vi "读取dev setup.vi"() -> (3 "输出簇":T1)   [LabVIEW 2011]
uses:
  <vilib>/Utility/config.llb/Read Key (Double).vi
  <vilib>/Utility/config.llb/Read Key (String).vi
  <vilib>/Utility/config.llb/Write Key (Double).vi
  <vilib>/Utility/config.llb/Write Key (String).vi
  <vilib>/Utility/config.llb/NI_LVConfig.lvlib
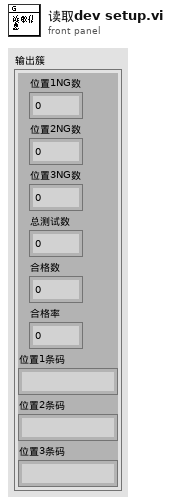
[diagram p1: front panel]
types:
  T1 = cluster{"位置1NG数 ":dbl, "位置2NG数 ":dbl, "位置3NG数 ":dbl, "总测试数":dbl, "合格数":dbl, "合格率":dbl, "位置1条码":string, "位置2条码":string, "位置3条码":string}
  T2 = typedef "NI_LVConfig.lvlib/Config Data RefNum.ctl" = refnum<k1>
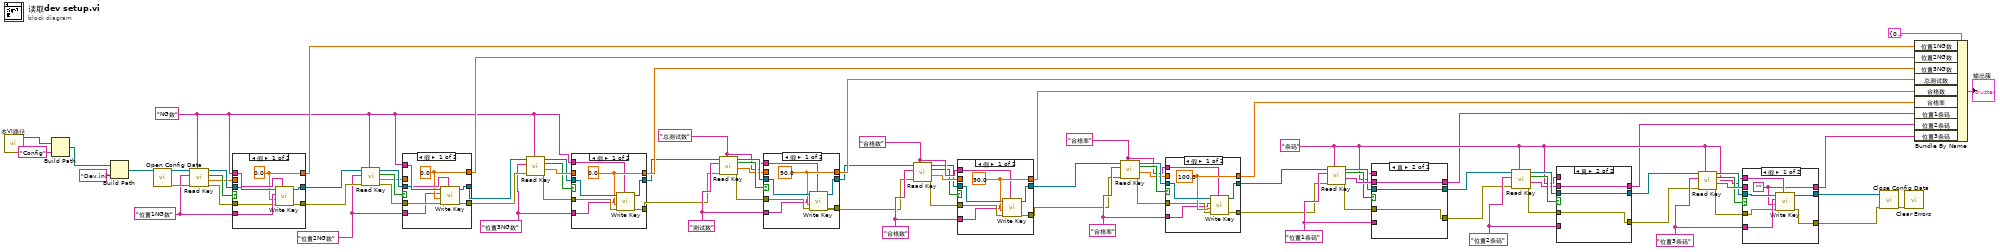
[diagram p0: block diagram]
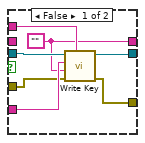
[diagram p3: hidden frame]
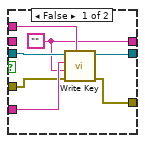
[diagram p4: hidden frame]
diagram:
  w11 = "位置3条码" ("开关名称")
  w22 = "位置2条码" ("开关名称")
  w8 = "条码" ("section")
  w25 = "位置1条码" ("开关名称")
  w37 = "合格数" ("section")
  w32 = "合格数" ("开关名称")
  w38 = "总测试数" ("section")
  w45 = "测试数" ("开关名称")
  w46 = "位置3NG数" ("开关名称")
  w48 = "NG数"
  w47 = "位置2NG数" ("开关名称")
  w64 = "位置1NG数" ("开关名称")
  w79 = "合格率" ("section")
  w84 = "合格率" ("开关名称")
  n1 = call "本VI路径.vi"() -> ("stripped path"=w69:path)  [unwired: 11 in]
  n2 = Build Path(base path=w69, name or relative path="Config" ("名称或相对路径")) -> (appended path=w85:path)
  n3 = Build Path(base path=w85, name or relative path="Dev.ini" ("名称或相对路径")) -> (appended path=w87:path)
  n4 = call <vilib>:"Open Config Data.vi"("configuration file path"=w87) -> ("error out"=w66:errorcluster, "refnum"=w67:T2)  [unwired: 8 in, 1 out]
  n5 = call-poly <vilib>:"Read Key.vi"("section"=w48, "error in (no error)"=w66, "key"=w64, "refnum"=w67) -> ("error out"=w61:errorcluster, "value"=w62:dbl, "found?"=w65:bool, "refnum out"=w63:T2)  [unwired: 4 in]
  n6 = case shown="假" w65 {
    tunnel: w63 -> [w94 w97]
    tunnel: w48 -> [w93 _]
    tunnel: w64 -> [w92 _]
    tunnel: [w91 w97] -> w60
    tunnel: [w90 w96] -> w75
    tunnel: w62 -> [_ w96]
    tunnel: [w88 w95] -> w56
    tunnel: w61 -> [w89 w95]
    frame False {
      w90 = 0.0 ("value")
      n7 = call-poly <vilib>:"Write Key.vi"("section"=w93, "error in (no error)"=w89, "value"=w90, "key"=w92, "refnum"=w94) -> ("error out"=w88:errorcluster, "refnum out"=w91:T2)  [unwired: 4 in, 1 out]
    }
    frame True {
    }
  }
  n8 = call-poly <vilib>:"Read Key.vi"("section"=w48, "error in (no error)"=w56, "key"=w47, "refnum"=w60) -> ("error out"=w57:errorcluster, "value"=w55:dbl, "found?"=w59:bool, "refnum out"=w58:T2)  [unwired: 4 in]
  n9 = case shown="假" w59 {
    tunnel: w58 -> [w104 w107]
    tunnel: w48 -> [w103 _]
    tunnel: [w102 w107] -> w50
    tunnel: [w101 w106] -> w74
    tunnel: w55 -> [_ w106]
    tunnel: [w99 w105] -> w49
    tunnel: w57 -> [w100 w105]
    tunnel: w47 -> [w98 _]
    frame False {
      w101 = 0.0 ("value")
      n10 = call-poly <vilib>:"Write Key.vi"("section"=w103, "error in (no error)"=w100, "value"=w101, "key"=w98, "refnum"=w104) -> ("error out"=w99:errorcluster, "refnum out"=w102:T2)  [unwired: 4 in, 1 out]
    }
    frame True {
    }
  }
  n11 = call-poly <vilib>:"Read Key.vi"("section"=w48, "error in (no error)"=w49, "key"=w46, "refnum"=w50) -> ("error out"=w53:errorcluster, "value"=w54:dbl, "found?"=w51:bool, "refnum out"=w52:T2)  [unwired: 4 in]
  n12 = case shown="假" w51 {
    tunnel: w52 -> [w114 w117]
    tunnel: [w113 w117] -> w39
    tunnel: [w112 w116] -> w73
    tunnel: w54 -> [_ w116]
    tunnel: [w110 w115] -> w40
    tunnel: w53 -> [w111 w115]
    tunnel: w48 -> [w109 _]
    tunnel: w46 -> [w108 _]
    frame False {
      w112 = 0.0 ("value")
      n13 = call-poly <vilib>:"Write Key.vi"("section"=w109, "error in (no error)"=w111, "value"=w112, "key"=w108, "refnum"=w114) -> ("error out"=w110:errorcluster, "refnum out"=w113:T2)  [unwired: 4 in, 1 out]
    }
    frame True {
    }
  }
  n14 = call-poly <vilib>:"Read Key.vi"("section"=w38, "error in (no error)"=w40, "key"=w45, "refnum"=w39) -> ("error out"=w42:errorcluster, "value"=w41:dbl, "found?"=w44:bool, "refnum out"=w43:T2)  [unwired: 4 in]
  n15 = case shown="假" w44 {
    tunnel: w43 -> [w124 w127]
    tunnel: [w123 w127] -> w31
    tunnel: [w122 w126] -> w72
    tunnel: w41 -> [_ w126]
    tunnel: [w120 w125] -> w30
    tunnel: w42 -> [w121 w125]
    tunnel: w38 -> [w119 _]
    tunnel: w45 -> [w118 _]
    frame False {
      w122 = 90.0 ("value")
      n16 = call-poly <vilib>:"Write Key.vi"("section"=w119, "error in (no error)"=w121, "value"=w122, "key"=w118, "refnum"=w124) -> ("error out"=w120:errorcluster, "refnum out"=w123:T2)  [unwired: 4 in, 1 out]
    }
    frame True {
    }
  }
  n17 = call-poly <vilib>:"Read Key.vi"("section"=w37, "error in (no error)"=w30, "key"=w32, "refnum"=w31) -> ("error out"=w35:errorcluster, "value"=w36:dbl, "found?"=w33:bool, "refnum out"=w34:T2)  [unwired: 4 in]
  n18 = case shown="假" w33 {
    tunnel: w34 -> [w134 w137]
    tunnel: [w133 w137] -> w77
    tunnel: [w132 w136] -> w71
    tunnel: w36 -> [_ w136]
    tunnel: [w130 w135] -> w78
    tunnel: w35 -> [w131 w135]
    tunnel: w37 -> [w129 _]
    tunnel: w32 -> [w128 _]
    frame False {
      w132 = 90.0 ("value")
      n19 = call-poly <vilib>:"Write Key.vi"("section"=w129, "error in (no error)"=w131, "value"=w132, "key"=w128, "refnum"=w134) -> ("error out"=w130:errorcluster, "refnum out"=w133:T2)  [unwired: 4 in, 1 out]
    }
    frame True {
    }
  }
  n20 = call-poly <vilib>:"Read Key.vi"("section"=w79, "error in (no error)"=w78, "key"=w84, "refnum"=w77) -> ("error out"=w81:errorcluster, "value"=w80:dbl, "found?"=w83:bool, "refnum out"=w82:T2)  [unwired: 4 in]
  n21 = case shown="假" w83 {
    tunnel: w82 -> [w144 w147]
    tunnel: [w143 w147] -> w23
    tunnel: [w142 w146] -> w70
    tunnel: w80 -> [_ w146]
    tunnel: [w140 w145] -> w24
    tunnel: w81 -> [w141 w145]
    tunnel: w79 -> [w139 _]
    tunnel: w84 -> [w138 _]
    frame False {
      w142 = 100.0 ("value")
      n22 = call-poly <vilib>:"Write Key.vi"("section"=w139, "error in (no error)"=w141, "value"=w142, "key"=w138, "refnum"=w144) -> ("error out"=w140:errorcluster, "refnum out"=w143:T2)  [unwired: 4 in, 1 out]
    }
    frame True {
    }
  }
  n23 = call-poly <vilib>:"Read Key.vi"("section"=w8, "error in (no error)"=w24, "key"=w25, "refnum"=w23) -> ("error out"=w28:errorcluster, "value"=w29:string, "found?"=w26:bool, "refnum out"=w27:T2)  [unwired: 4 in]
  n24 = case shown="真" w26 {
    tunnel: w27 -> [w154 w157]
    tunnel: [w151 w157] -> w16
    tunnel: w29 -> [_ w155]
    tunnel: [w150 w156] -> w17
    tunnel: w28 -> [w149 w156]
    tunnel: w8 -> [w152 _]
    tunnel: w25 -> [w153 _]
    tunnel: [w148 w155] -> w4
    frame False {
      w148 = ""
      n25 = call-poly <vilib>:"Write Key.vi"("section"=w152, "error in (no error)"=w149, "value"=w148, "key"=w153, "refnum"=w154) -> ("error out"=w150:errorcluster, "refnum out"=w151:T2)  [unwired: 4 in, 1 out]
    }
    frame True {
    }
  }
  n26 = call-poly <vilib>:"Read Key.vi"("section"=w8, "error in (no error)"=w17, "key"=w22, "refnum"=w16) -> ("error out"=w19:errorcluster, "value"=w18:string, "found?"=w21:bool, "refnum out"=w20:T2)  [unwired: 4 in]
  n27 = case shown="真" w21 {
    tunnel: w20 -> [w164 w167]
    tunnel: [w161 w167] -> w9
    tunnel: w18 -> [_ w165]
    tunnel: [w160 w166] -> w10
    tunnel: w19 -> [w159 w166]
    tunnel: w8 -> [w162 _]
    tunnel: w22 -> [w163 _]
    tunnel: [w158 w165] -> w3
    frame False {
      w158 = ""
      n28 = call-poly <vilib>:"Write Key.vi"("section"=w162, "error in (no error)"=w159, "value"=w158, "key"=w163, "refnum"=w164) -> ("error out"=w160:errorcluster, "refnum out"=w161:T2)  [unwired: 4 in, 1 out]
    }
    frame True {
    }
  }
  n29 = call-poly <vilib>:"Read Key.vi"("section"=w8, "error in (no error)"=w10, "key"=w11, "refnum"=w9) -> ("error out"=w14:errorcluster, "value"=w15:string, "found?"=w12:bool, "refnum out"=w13:T2)  [unwired: 4 in]
  n30 = case shown="假" w12 {
    tunnel: w13 -> [w174 w177]
    tunnel: [w171 w177] -> w6
    tunnel: w15 -> [_ w175]
    tunnel: [w170 w176] -> w7
    tunnel: w14 -> [w169 w176]
    tunnel: w8 -> [w172 _]
    tunnel: w11 -> [w173 _]
    tunnel: [w168 w175] -> w2
    frame False {
      w168 = ""
      n31 = call-poly <vilib>:"Write Key.vi"("section"=w172, "error in (no error)"=w169, "value"=w168, "key"=w173, "refnum"=w174) -> ("error out"=w170:errorcluster, "refnum out"=w171:T2)  [unwired: 4 in, 1 out]
    }
    frame True {
    }
  }
  n32 = call <vilib>:"Close Config Data.vi"("error in (no error)"=w7, "refnum"=w6) -> ("error out"=w76:errorcluster)  [unwired: 8 in, 1 out]
  n33 = call <vilib>:"Clear Errors.vi"("error in (no error)"=w76) -> ()  [unwired: 6 in, 1 out]
  n34 = Bundle By Name(cluster=T1 {"位置1NG数 "=0.0, "位置2NG数 "=0.0, "位置3NG数 "=0.0, "总测试数"=0.0, "合格数"=0.0, "合格率"=0.0, "位置1条码"="", "位置2条码"="", "位置3条码"=""}, "位置1NG数"=w75, "位置2NG数"=w74, "位置3NG数"=w73, "总测试数"=w72, "合格数"=w71, "合格率"=w70, "位置1条码"=w4, "位置2条码"=w3, "位置3条码"=w2) -> (→"输出簇":T1)
